vi "Create All Message Queues.vi"(8 "error in (no error)":errorcluster) -> (0 "error out":errorcluster, 3 "Message Queues out":T1)   [LabVIEW 2015, in "Message Queue.lvlib"]
doc: "This VI creates and initializes all the message queues for your application. If your application requires more than one message queue, right-click the \"Message Queues\" constant above and select Open Type Def. Add the new Message Queue(s) to the type definition, then initialize them in this VI."
uses:
  Message Queue.lvlib
  All Message Queues.ctl
  Message Cluster.ctl
  Enqueue Message (Single).vi
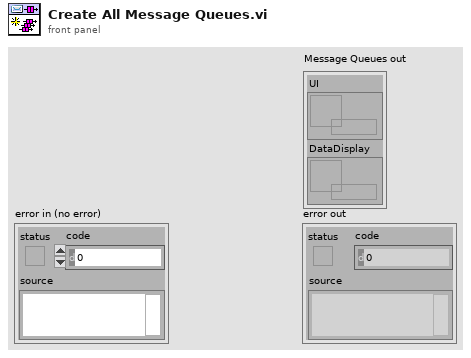
[diagram p1: front panel]
types:
  T1 = typedef "Message Queue.lvlib/All Message Queues.ctl" = cluster{"UI":refnum<queue>, "DataDisplay":refnum<queue>}
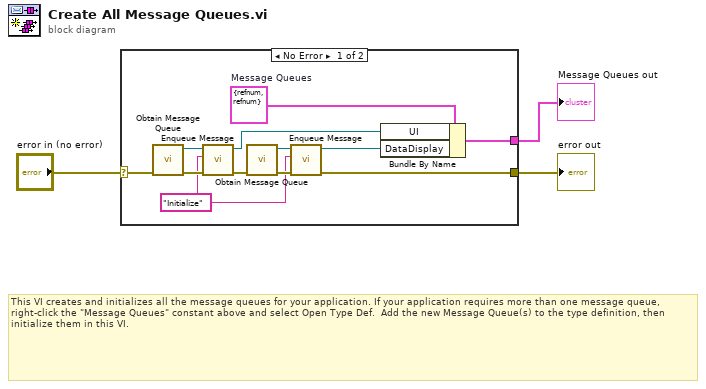
[diagram p0: block diagram]
diagram:
  # "This VI creates and initializes all the message queues for your application. If your application requires more than one message queue, right-click the \"Message Queues\" constant above and select Open Type Def.  Add the new Message Queue(s) to the type definition, then initialize them in this VI."
  n1 = case shown="No Error" "error in (no error)" {
    selector: "error in (no error)" -> [w13 w16]
    tunnel: [w5 w16] -> w3
    tunnel: [w14 _] -> w2
    frame No Error {
      w4 = "Initialize" ("Message")
      w15 = T1 {"UI"=refnum, "DataDisplay"=refnum}  # Message Queues
      n2 = call "Obtain Message Queue.vi"("error in (no error)"=w13) -> ("error out"=w10:errorcluster, "Message Queue"=w12:refnum<queue>)  [unwired: 9 in]
      n3 = call-poly "Enqueue Message.vi"("error in (no error)"=w10, "Message"=w4, "Message Queue"=w12) -> ("error out"=w11:errorcluster, "dup Message Queue"=w7:refnum<queue>)  [unwired: 7 in]
      n4 = call "Obtain Message Queue.vi"("error in (no error)"=w11) -> ("error out"=w6:errorcluster, "Message Queue"=w9:refnum<queue>)  [unwired: 9 in]
      n5 = call-poly "Enqueue Message.vi"("error in (no error)"=w6, "Message"=w4, "Message Queue"=w9) -> ("error out"=w5:errorcluster, "dup Message Queue"=w8:refnum<queue>)  [unwired: 7 in]
      n6 = Bundle By Name(cluster=w15, "UI"=w7, "DataDisplay"=w8) -> (w14:T1)
    }
    frame Error {
    }
  }
  "Message Queues out" <- w2
  "error out" <- w3
